vi "Get Actuals.vi"(8 "error in (no error)":errorcluster, 11 "input cluster":T1={"Session_Control"="Sess_Control", "Session_Params"="Sess_Params", "Session_Actuals"="Sess_Actuals", "Session_Acknowledge"="Sess_Ack", "Session_H2_Sensor"="H2_Sensor_Session", "Session_DILICO_MeasurementRequest"="Session_DILICO_MeasurementRequest", "Session_DILICO_Voltages"="Session_DILICO_Voltages"}) -> (0 "error out":errorcluster, 2 "Actual Values":map{string, dbl}(c390), 3 "output cluster":T1={"Session_Control"="Session_Control", "Session_Params"="Session_Params", "Session_Actuals"="Session_Actuals", "Session_Acknowledge"="Session_Acknowledge", "Session_H2_Sensor"="H2_Sensor_Session", "Session_DILICO_MeasurementRequest"="Session_DILICO_MeasurementRequest", "Session_DILICO_Voltages"="Session_DILICO_Voltages"})   [LabVIEW 2025, in "phlair-busch-can-bus.lvlib"]
uses:
  phlair-busch-can-bus.lvlib
  CAN Frame Sessions.ctl
  <vilib>/xnet/xnet.llb/XNET Read (Signal Single-point).vi
  <resource>/objmgr/xnet.rc
panel:
  out "Array 2":u32[](array[numeric])
  out "Array":dbl[](array[numeric])
  out "data":dbl[](array[numeric]) format="%.2f"
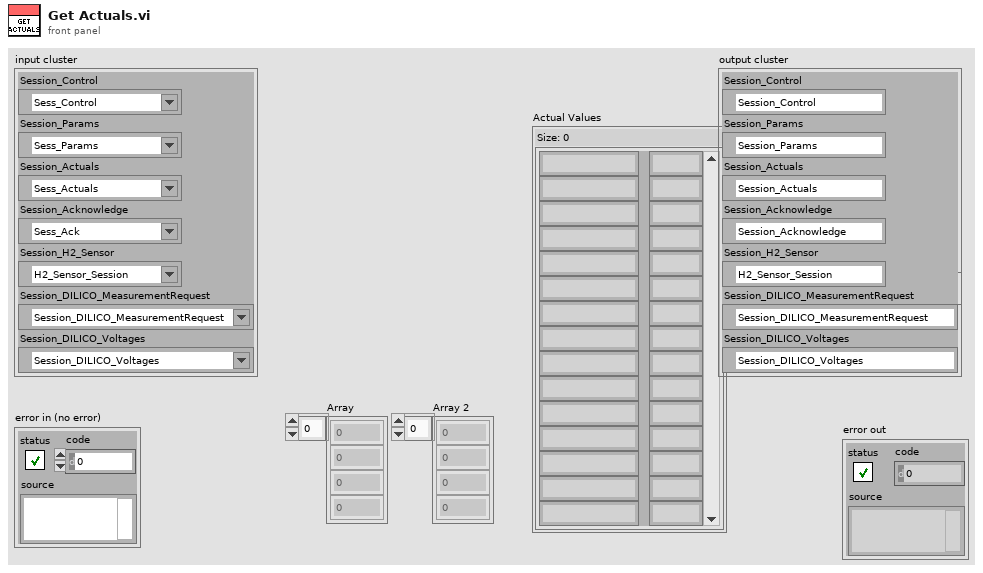
[diagram p1: front panel]
types:
  T1 = typedef "phlair-busch-can-bus.lvlib/CAN Frame Sessions.ctl" = cluster{"Session_Control":refnum<k21>, "Session_Params":refnum<k21>, "Session_Actuals":refnum<k21>, "Session_Acknowledge":refnum<k21>, "Session_H2_Sensor":refnum<k21>, "Session_DILICO_MeasurementRequest":refnum<k21>, "Session_DILICO_Voltages":refnum<k21>}
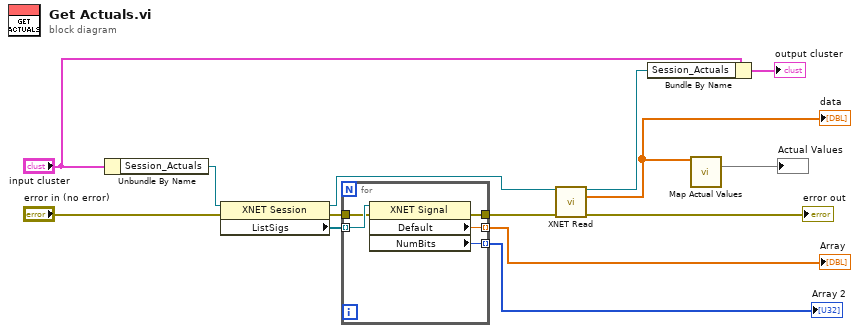
[diagram p0: block diagram]
diagram:
  n1 = Unbundle By Name("input cluster") -> ("Session_Actuals"=w5:refnum<k21>)
  n2 = property class="XNET Session"(reference=w5, error in="error in (no error)") -> (reference out=w4:refnum<k21>, error out=w2:errorcluster, "ListSigs"=w8:refnum<k21>[])
  n3 = for {
    tunnel: w8 -> [w19] mode=indexing
    tunnel: [w18] -> w7 mode=indexing
    tunnel: [w17] -> w6 mode=indexing
    tunnel: w2 -> [w16]
    tunnel: [w15] -> w1
    n4 = property class="XNET Signal"(reference=w19, error in=w16) -> (error out=w15:errorcluster, "Default"=w18:dbl, "NumBits"=w17:u32)  [unwired: 1 out]
  }
  "Array" <- w7
  "Array 2" <- w6
  n5 = call-poly <vilib>:"XNET Read.vi"("session in"=w4, "error in (no error)"=w1) -> ("session out"=w12:refnum<k21>, "data"=w9:dbl[], "error out"=→"error out":errorcluster)  [unwired: 11 in]
  "data" <- w9
  n6 = Bundle By Name(cluster="input cluster", "Session_Actuals"=w12) -> (→"output cluster":T1)
  n7 = call "Map Actual Values.vi"("Actual Values Array In"=w9) -> ("Actual Values"=→"Actual Values":map{string, dbl})  [unwired: 12 in, 2 out]
